vi "Actor Core.vi"(8 "error in":errorcluster, 11 "Mag Lab Measure Base in":refnum<class "Mag Lab Measure Base.lvclass">) -> (0 "error out":errorcluster, 3 "Actor out":refnum<class "Actor.lvclass">)   [LabVIEW 2015, in "Mag Lab Measure Base.lvclass"]
doc: "(<B>Filename</B>: Actor Framework.lvlib:Actor.lvclass:Actor Core.vi)\n\nReceives messages to the actor, reacts to them, and initiates any error handling that may shut the actor down.\n\nDescendant classes may override this VI to append parallel tasks for the actor to complete while it handles messages. Overrides use the Call Parent Method node."
uses:
  Mag Lab Measure Base.lvclass
  <vilib>/ActorFramework/Actor/Actor.lvclass
  Mag Lab Graph/MagLabGraph.lvclass
  Mag Lab Root/Mag Lab Root.lvclass/Mag Lab Root.ctl
  Mag Lab Measure Base.lvclass/Mag Lab Measure Base.ctl
  <vilib>/ActorFramework/Actor/Actor.lvclass/Actor.ctl
  <vilib>/ActorFramework/Message Enqueuer/Message Enqueuer.lvclass/Message Enqueuer.ctl
  Mag Lab Measure Base Messages/Open sub-object parameters Msg/Open nested object parameters Msg.lvclass/Open nested object parameters Msg.ctl
  <vilib>/ActorFramework/Message Enqueuer/Init from Existing Queue.vi
  <vilib>/ActorFramework/Message Enqueuer/Enqueue.vi
  <vilib>/ActorFramework/Message Priority Queue/Priority Enqueue.vi
  <vilib>/ActorFramework/Message Enqueuer/Message Enqueuer.lvclass
  Mag Lab Root Messages/Close Front Panel Msg/Close Front Panel Msg.lvclass
  Mag Lab Measure Base Messages/Open sub-object parameters Msg/Open nested object parameters Msg.lvclass
  Mag Lab Root/Mag Lab Root.lvclass
  Mag Lab Error Handler/Mag Lab Error Handler.lvclass
panel:
  in  "No UI has been defined for this \nobject":bool
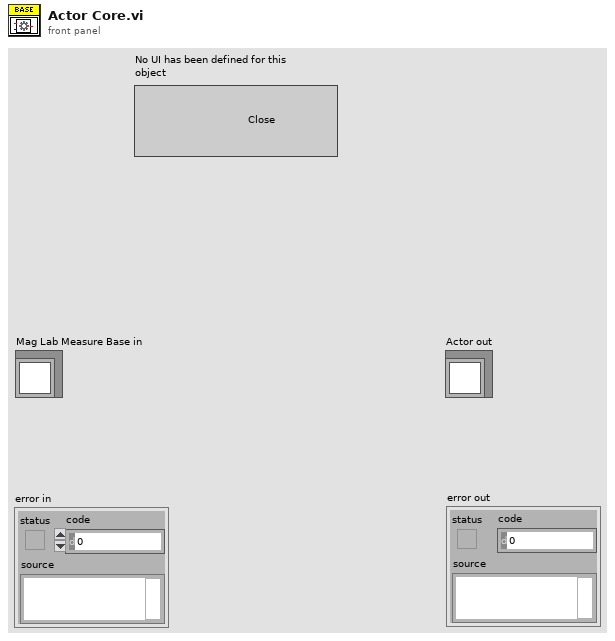
[diagram p1: front panel]
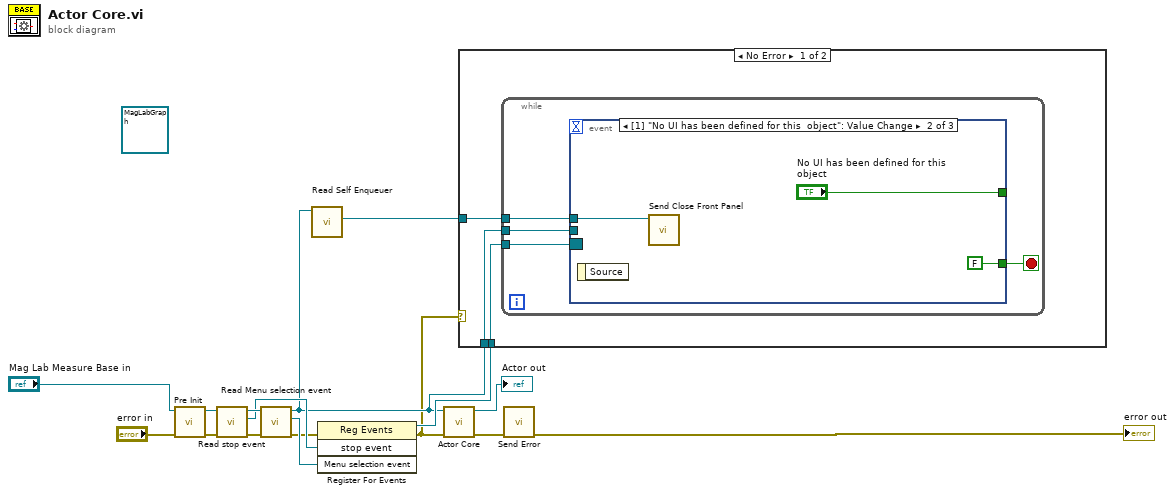
[diagram p0: block diagram]
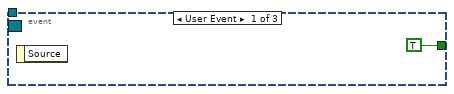
[diagram p2: hidden frame]
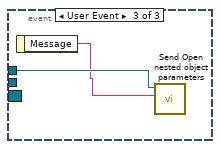
[diagram p3: hidden frame]
diagram:
  (unwired) refnum<class "MagLabGraph.lvclass"> refnum ("MagLabGraph.lvclass")
  n1 = call-dynamic "Pre Init.vi"("error in (no error)"="error in", "Mag Lab Measure Base in"="Mag Lab Measure Base in") -> ("error out"=w6:errorcluster, "Mag Lab Measure Base out"=w11:refnum<class "Mag Lab Measure Base.lvclass">)  [unwired: 8 in]
  n2 = call "Read stop event.vi"("error in (no error)"=w6, "Mag Lab Root in"=w11) -> ("error out"=w5:errorcluster, "stop event"=w9:refnum<user-event>, "Mag Lab Root out"=w10:refnum<class "Mag Lab Measure Base.lvclass">)  [unwired: 7 in]
  n3 = call "Read Menu selection event.vi"("error in (no error)"=w5, "Mag Lab Measure Base in"=w10) -> ("error out"=w4:errorcluster, "Menu selection event"=w8:refnum<user-event>, "Mag Lab Measure Base out"=w7:refnum<class "Mag Lab Measure Base.lvclass">)  [unwired: 7 in]
  n4 = call <vilib>:"Read Self Enqueuer.vi"("Actor"=w7) -> ("Self Enqueuer"=w13:refnum<class "Message Enqueuer.lvclass">)  [unwired: 10 in]
  n5 = register-events(error in=w4, w9, w8) -> (reference out=w12:refnum<event-registration>, error out=w1:errorcluster)  [unwired: 1 in]
  n6 = call-parent "Actor Core.vi"("error in"=w1, "Actor in"=w7) -> ("error out"=w3:errorcluster, "Actor out"=→"Actor out":refnum<class "Actor.lvclass">)  [unwired: 8 in]
  n7 = case shown="No Error" w1 {
    tunnel: w13 -> [w19 _]
    tunnel: w12 -> [w18 _]
    tunnel: w7 -> [w17 _]
    frame No Error {
      n8 = while {
        tunnel: w18 -> [w22]
        tunnel: w19 -> [w21]
        tunnel: w17 -> [w20]
        stop <- w23 stop-if-true
        n9 = event shown="[1] \"No UI has been defined for this  object\": Value Change" {
          selector: w22 -> [_ _ _]
          dyn-events: _ -> [_ _ _]
          timeout: _ -> [_ _ _]
          tunnel: [TRUE FALSE _] -> w23
          tunnel: w21 -> [_ w25 w29]
          tunnel: w20 -> [_ _ _]
          tunnel: [_ "No UI has been defined for this \nobject" _] -> _
          event User Event {
            n10 = event-data() -> ()  [unwired: 1 in, 1 out]
          }
          event "No UI has been defined for this \nobject": Value Change {
            n11 = event-data() -> ()  [unwired: 1 in, 1 out]
            n12 = call "Send Close Front Panel.vi"("Message Enqueuer"=w25) -> ()  [unwired: 9 in, 2 out]
          }
          event User Event {
            n13 = event-data() -> ("Message"=w28:string)  [unwired: 1 in]
            n14 = call "Send Open nested object parameters.vi"("Object name"=w28, "Message Enqueuer"=w29) -> ()  [unwired: 8 in, 2 out]
          }
        }
      }
    }
    frame Error {
    }
  }
  n15 = call "Send Error.vi"("error in (no error)"=w3) -> ("error out"=→"error out":errorcluster)  [unwired: 9 in, 1 out]
